vi "Public Key Memory Authentication.vi"(7 "Keys":cluster{"Private":string, "Public":string}, 8 "Error In":errorcluster, 9 "Passphrase":string, 10 "Username":string, 11 "Session In":refnum<class "Session.lvclass">) -> (0 "Error Out":errorcluster, 3 "Sesssion Out":refnum<class "Session.lvclass">)   [LabVIEW 2018, in "Toolkit.lvlib" / "Session.lvclass"]
doc: "Authenticate this session for a user using a public-private key pair as binary data."
uses:
  Session.lvclass
  Session.lvclass/Session.ctl
  SSH/SSH.lvclass/SSH.ctl
  Toolkit.lvlib
  SSH/SSH.lvclass
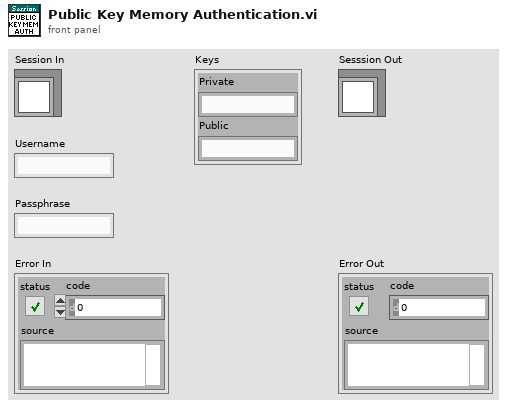
[diagram p1: front panel]
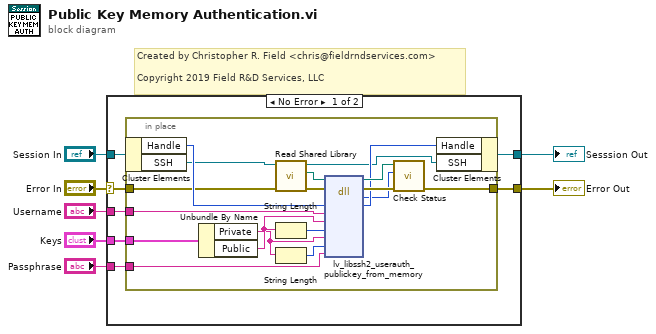
[diagram p0: block diagram]
diagram:
  # "Created by Christopher R. Field <chris@fieldrndservices.com>\n\nCopyright 2019 Field R&D Services, LLC"
  n1 = case shown="No Error" "Error In" {
    selector: "Error In" -> [w11 w34]
    tunnel: [w13 w34] -> w6
    tunnel: "Session In" -> [w12 w33]
    tunnel: [w14 w33] -> w4
    tunnel: "Username" -> [w10 _]
    tunnel: "Passphrase" -> [w9 _]
    tunnel: "Keys" -> [w8 _]
    frame No Error {
      n2 = in-place {
        in-place-border: [w30] -> w13
        in-place-border: w11 -> [w26]
        in-place-border: w10 -> [w25]
        in-place-border: w9 -> [w24]
        in-place-border: w8 -> [w23]
        n3 = in-place-cluster #1(w12) -> ("Handle"=w29:u64, "SSH"=w17:refnum<class "SSH.lvclass">)
        n4 = Unbundle By Name(w23) -> ("Private"=w20:string, "Public"=w21:string)
        n5 = call "Read Shared Library.vi"("Error In"=w26, "SSH In"=w17) -> ("Error Out"=w18:errorcluster, "lv-libssh2 Shared Library"=w15:path, "SSH Out"=w16:refnum<class "SSH.lvclass">)  [unwired: 7 in]
        n6 = String Length(string=w21) -> (length=w22:i32)
        n7 = String Length(string=w20) -> (length=w19:i32)
        n8 = dll-call lib="D:/Users/cfield/Code/Field R&D Services/SSH/LV-LIBSSH2/LabVIEW/trunk/src/Toolkit/Support/lv-libssh2.*" fn="lv_libssh2_userauth_publickey_from_memory"(path in=w15, error in=w18, "session"=w29, "username"=w25, "public_key_data"=w21, "public_key_data_len"=w22, "private_key_data"=w20, "private_key_data_len"=w19, "passphrase"=w24) -> (path out=w32:path, error out=w31:errorcluster, "result"=w27:i32, "session"=w28:u64)  [unwired: 7 in]
        n9 = call "Check Status.vi"("Error In"=w31, "Status"=w27, "lv-libssh2 Shared Library In"=w32) -> ("Error Out"=w30:errorcluster)  [unwired: 7 in, 1 out]
        n10 = in-place-cluster #1("Handle"=w28, "SSH"=w16) -> (w14:refnum<class "Session.lvclass">)
      }
    }
    frame Error {
    }
  }
  "Sesssion Out" <- w4
  "Error Out" <- w6
